vi "DataReceiver.vi"() -> ()   [LabVIEW 2014]
doc: "This VI in conjunction with Target Fullness.vi demonstrates how to use network streams properties to determine how effectively data is being delivered through the network stream before it becomes congested and has to block before accepting new data. Setting the writer wait time smaller than the reader wait time will cause the reader and writer to gradually fill up. In this situation, the reader is the bottleneck of the transfer. Setting the reader wait time smaller than the writer wait time will cause the reader and writer to gradually empty. In this situation, the writer is the bottleneck of the transfer.\n\n<B>Note:</B> Requires Target Fullnes.vi located in the same directory as this VI."
uses:
  <resource>/objmgr/ni.dex.rc
panel:
  out "Numeric":i32
  out "Waveform Chart":waveform(dbl)[](graph)
  in  "Target IP Address":string="localhost"
  in  "Scale":dbl=7.38e-11
  in  "Spacing":dbl=0.002
  out "error out":errorcluster
  in  "Reader Wait Time":u32=25
  in  "stop":bool
  out "Elements in Reader":i32(slide) scale=0.0..100.0
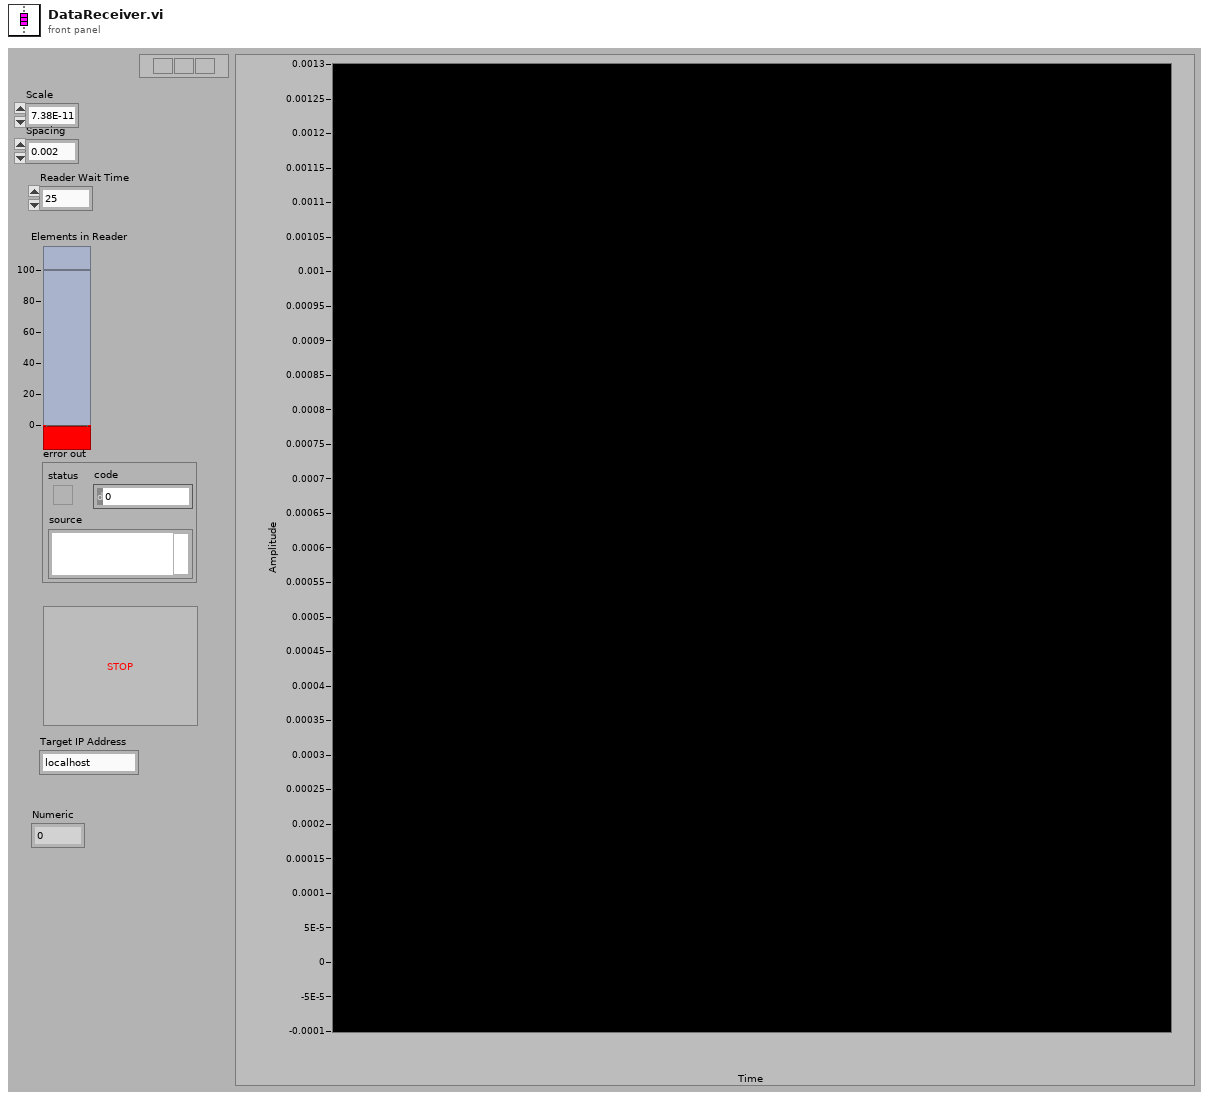
[diagram p1: front panel]
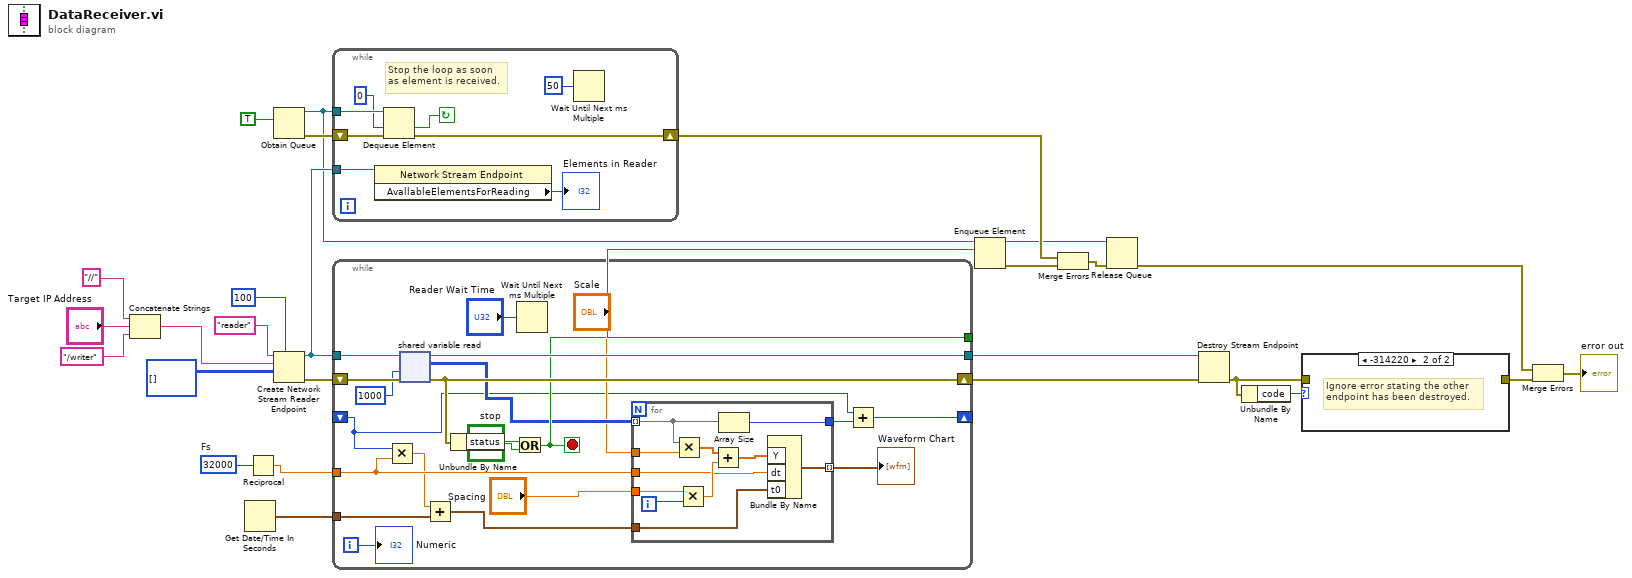
[diagram p0: block diagram]
diagram:
  w7 = 32000  # Fs
  n1 = Concatenate Strings("//" ("reader url"), "Target IP Address", "/writer" ("string")) -> (w1:string)
  n2 = Get Date/Time In Seconds() -> (seconds since 1Jan1904=w5:timestamp)
  n3 = Reciprocal(x=w7) -> (1/x=w6:dbl)
  n4 = Obtain Queue(element data type=TRUE ("stop")) -> (queue out=w15:refnum<queue>, error out=w20:errorcluster)  [unwired: 4 in, 1 out]
  n5 = Create Network Stream Reader Endpoint(7:100 ("reader buffer size"), 9:i32[][] [], 10:w1, 11:"reader" ("writer name")) -> (0:w26:errorcluster, 3:w23:refnum<k21>)  [unwired: 3 in]
  n6 = while {
    tunnel: w23 -> [w35]
    tunnel: w15 -> [w32]
    shift-right: [w30] -> w22
    shift-left: w20 -> [w29]
    stop <- w28 continue-if-true
    # "Stop the loop as soon \nas element is received."
    n7 = property class="Network Stream Endpoint"(reference=w35) -> ("AvallableElementsForReading"=→"Elements in Reader":i32)  [unwired: 1 in, 2 out]
    n8 = Dequeue Element(queue=w32, timeout in ms (-1)=0, error in (no error)=w29) -> (timed out?=w28:bool, error out=w30:errorcluster)  [unwired: 2 out]
    n9 = Wait Until Next ms Multiple(millisecond multiple=u32 50 ("milliseconds to wait")) -> ()  [unwired: 1 out]
  }
  n10 = while {
    tunnel: w23 -> [w55]
    tunnel: [w54] -> w25
    shift-right: [w49] -> w24
    shift-left: w26 -> [w56]
    tunnel: [w48] -> w12
    shift-right: [w45] -> _
    shift-left: _ -> [w38]
    tunnel: w6 -> [w42]
    tunnel: w5 -> [w40]
    i -> [w36]
    stop <- w48 stop-if-true
    n11 = Multiply(x=w38, y=w42) -> (x*y=w41:dbl)
    n12 = shared-variable-read(w55, w56, 1000 ("timeout in ms (-1)")) -> (w54:refnum<k21>, w49:errorcluster, w47:i32[][])  [unwired: 1 out]
    n13 = Add(x=w41, y=w40) -> (x+y=w39:timestamp)
    n14 = Unbundle By Name(w49) -> ("status"=w50:bool)
    n15 = Or(x=w50, y="stop") -> (x .or. y?=w48:bool)
    n16 = Wait Until Next ms Multiple(millisecond multiple="Reader Wait Time") -> ()  [unwired: 1 out]
    n17 = for {
      tunnel: w47 -> [w66] mode=indexing
      tunnel: [w67] -> w46
      tunnel: "Scale" -> [w65]
      tunnel: "Spacing" -> [w62]
      tunnel: w42 -> [w59]
      tunnel: w39 -> [w58]
      tunnel: [w57] -> w37 mode=indexing
      i -> [w63]
      n18 = Multiply(x=w66, y=w65) -> (x*y=w64:dbl[])
      n19 = Multiply(x=w62, y=w63) -> (x*y=w61:dbl)
      n20 = Add(x=w64, y=w61) -> (x+y=w60:dbl[])
      n21 = Array Size(array=w66) -> (size(s)=w67:i32)
      n22 = Bundle By Name("Y"=w60, "dt"=w59, "t0"=w58) -> (w57:waveform(dbl))  [unwired: 1 in]
    }
    "Waveform Chart" <- w37
    n23 = Add(x=w38, y=w46) -> (x+y=w45:i32)
    "Numeric" <- w36
  }
  n24 = Enqueue Element(queue=w15, element=w12) -> (queue out=w16:refnum<queue>, error out=w17:errorcluster)  [unwired: 2 in, 1 out]
  n25 = Merge Errors(w22, w17) -> (w19:errorcluster)
  n26 = Release Queue(queue=w16, error in (no error)=w19) -> (error out=w10:errorcluster)  [unwired: 1 in, 2 out]
  n27 = Destroy Stream Endpoint(8:w24, 11:w25) -> (0:w13:errorcluster)
  n28 = Unbundle By Name(w13) -> ("code"=w14:i32)
  n29 = case shown="-314220" w14 {
    tunnel: w13 -> [w68 _]
    tunnel: [w68 _] -> w11
    frame 0, Default {
    }
    frame -314220 {
      # "Ignore error stating the other\nendpoint has been destroyed."
    }
  }
  n30 = Merge Errors(w10, w11) -> (→"error out":errorcluster)
